vi "Sub_ArrayToString.vi"(10 "区切り文字":string="-", 11 "文字列配列":string[](array[string])=["a", "b", "c"]) -> (3 "結果文字列":string="a-b-c")   [LabVIEW 2018]
panel:
  # "<機能>\n　文字列配列を区切り文字で区切た文字列にする"
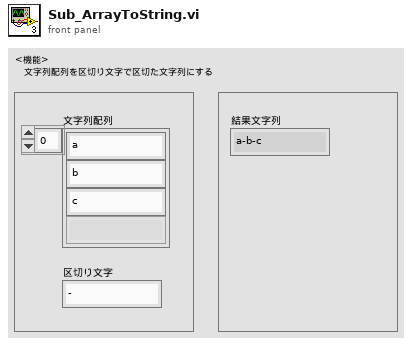
[diagram p1: front panel]
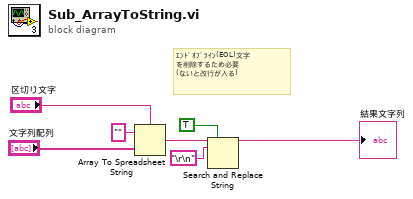
[diagram p0: block diagram]
diagram:
  # "ｴﾝﾄﾞｵﾌﾞﾗｲﾝ(EOL)文字\nを削除するため必要\n(ないと改行が入る)"
  n1 = Array To Spreadsheet String(delimiter (Tab)="区切り文字", array="文字列配列", 3:"" ("形式文字列")) -> (spreadsheet string=w3:string)
  n2 = Search and Replace String(replace all?=TRUE ("すべて置換?（F）"), input string=w3, search string="\r\n") -> (result string=→"結果文字列":string)  [unwired: 5 in, 3 out]
